vi "Cluster Gain and Phase.vi"(1 "Response":T1[](array[typedef]) {"Freq" format="%#.2f"; "Offset" format="%.3f"; "Gain" format="%.2f"; "Phase" format="%.1f"}, 2 "Stimulus":T1[](array[typedef]) {"Freq" format="%#.2f"; "Offset" format="%.3f"; "Gain" format="%.2f"; "Phase" format="%.1f"}) -> (0 "Gain and Phase out":T2 {"Phase SD" format="%.1f"; "Phase" format="%.1f"; "Gain SD" format="%.2f"; "Gain" format="%.2f"})   [LabVIEW 2016]
uses:
  Typedef - Gain and Phase.ctl
  Typedef - Sinusoidal Fit Coefficients.ctl
  comm/nan operations/nan operations.lvlib
panel:
  # "Gain:"
  # "+/-"
  # "Phase:"
  # "+/-"
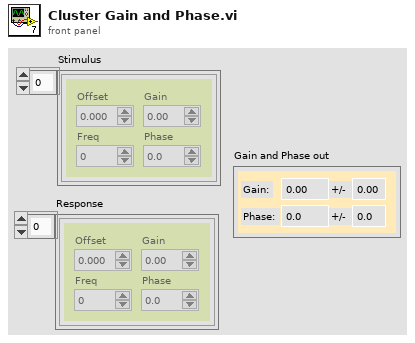
[diagram p1: front panel]
types:
  T1 = typedef "Typedef - Sinusoidal Fit Coefficients.ctl" = cluster{"Offset":dbl, "Gain":dbl, "Phase":dbl, "Freq":dbl}
  T2 = typedef "Typedef - Gain and Phase.ctl" = cluster{"Gain":dbl, "Gain SD":dbl, "Phase":dbl, "Phase SD":dbl}
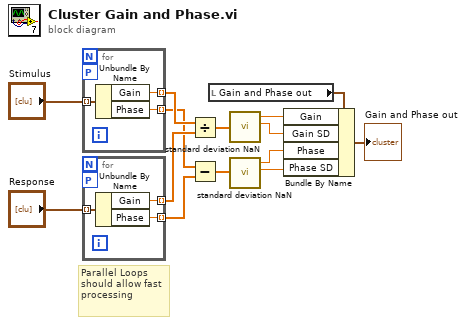
[diagram p0: block diagram]
diagram:
  # "Parallel Loops should allow fast processing"
  n1 = for {
    workers-P: _ -> [_]
    tunnel: "Stimulus" -> [w17] mode=indexing
    tunnel: [w16] -> w12 mode=indexing
    tunnel: [w15] -> w10 mode=indexing
    n2 = Unbundle By Name(w17) -> ("Gain"=w16:dbl, "Phase"=w15:dbl)
  }
  n3 = for {
    workers-P: _ -> [_]
    tunnel: "Response" -> [w20] mode=indexing
    tunnel: [w19] -> w11 mode=indexing
    tunnel: [w18] -> w9 mode=indexing
    n4 = Unbundle By Name(w20) -> ("Gain"=w19:dbl, "Phase"=w18:dbl)
  }
  n5 = Divide(x=w12, y=w11) -> (x/y=w8:dbl[])
  n6 = Subtract(x=w10, y=w9) -> (x-y=w7:dbl[])
  n7 = local read "Gain and Phase out"() -> (w6:T2)
  n8 = call "standard deviation NaN.vi"("Array"=w8) -> ("standard deviation"=w3:dbl, "mean"=w4:dbl)  [unwired: 2 in, 1 out]
  n9 = call "standard deviation NaN.vi"("Array"=w7) -> ("standard deviation"=w1:dbl, "mean"=w2:dbl)  [unwired: 2 in, 1 out]
  n10 = Bundle By Name(cluster=w6, "Gain"=w4, "Gain SD"=w3, "Phase"=w2, "Phase SD"=w1) -> (→"Gain and Phase out":T2)
